vi "Is This Control Of LabVIEW Object Class.vi"(8 "error in (no error)":errorcluster, 11 "Ctl Refnum":refnum<vi>) -> (0 "error out":errorcluster, 1 "Is this control of LabVIEW Object class?":bool, 3 "Ctl Refnum out":refnum<vi>)   [LabVIEW 2020]
doc: "Given a control refnum, this VI determines whether the control is a control of the LabVIEW class \"LabVIEW Object\". LabVIEW Object is the ancestor class of all other LabVIEW classes. This VI will return true for the regular class controls/indicators and for XControls whose type is LabVIEW Object.\n\nThis VI will return a \"not supported\" error in built applications."
uses:
  <vilib>/Utility/Data Type/NI_Data Type.lvlib
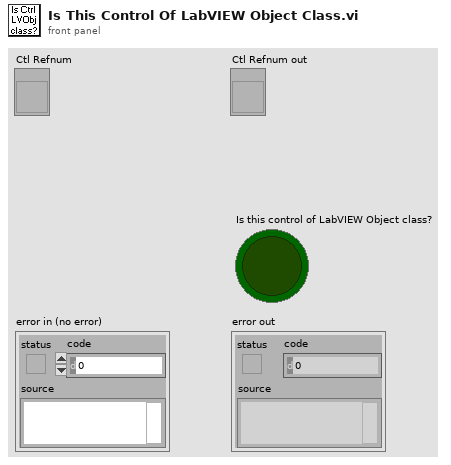
[diagram p1: front panel]
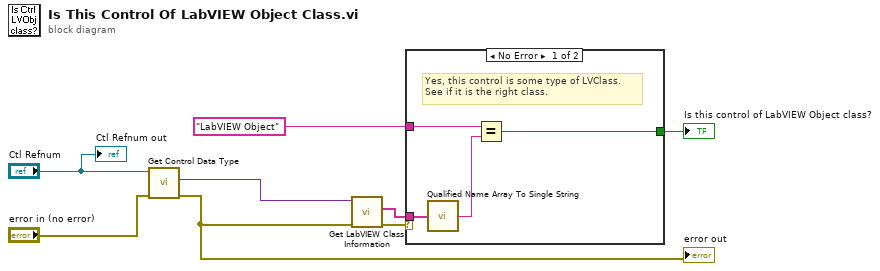
[diagram p0: block diagram]
diagram:
  n1 = call <vilib>:"Get Control Data Type.vi"("error in (no error)"="error in (no error)", "Control Refnum in"="Ctl Refnum") -> ("error out"=w3:errorcluster, "Control's Data Type"=w4:variant)  [unwired: 3 in, 1 out]
  "error out" <- w3
  n2 = call <vilib>:"Get LabVIEW Class Information.vi"("error in (no error)"=w3, "variant"=w4) -> ("error out"=w6:errorcluster, "qualified LabVIEW class name"=w7:string[])  [unwired: 7 in, 1 out]
  n3 = case shown="No Error" w6 {
    tunnel: w7 -> [w12 _]
    tunnel: [w10 _] -> w8
    tunnel: "LabVIEW Object" ("x") -> [w9 _]
    frame No Error {
      # "Yes, this control is some type of LVClass. \nSee if it is the right class."
      n4 = call <vilib>:"Qualified Name Array To Single String.vi"("Fully Qualified Array"=w12) -> ("Fully Qualified String"=w11:string)
      n5 = Equal?(x=w9, y=w11) -> (x = y?=w10:bool)
    }
    frame Error {
      # "Don't propagate this error. An error generated here just means the control is not an LVClass control."
    }
  }
  "Is this control of LabVIEW Object class?" <- w8
  "Ctl Refnum out" <- "Ctl Refnum"
